vi "Refresh Main Page Listboxes.vi"(6 "Main Page refnums":T3, 8 "error in (no error)":errorcluster, 9 "bitfile listbox":T1, 10 "APU listbox":T1, 11 "Item Ref in":T2 format="%.0x") -> (0 "error out":errorcluster, 1 "bitfile listbox out":T1, 2 "APU listbox out":T1, 3 "Item Ref out":T2=18446744073709551615 format="%.0x")   [LabVIEW 2020, in "Engine Simulation Toolkit System Explorer.lvlib"]
uses:
  Engine Simulation Toolkit System Explorer.lvlib
  Listbox State.ctl
  Main Page refnums.ctl
  <vilib>/NI VeriStand/Custom Device API/Custom Device Item Ref.ctl
  <vilib>/NI VeriStand/Custom Device API/Custom Device API.lvlib
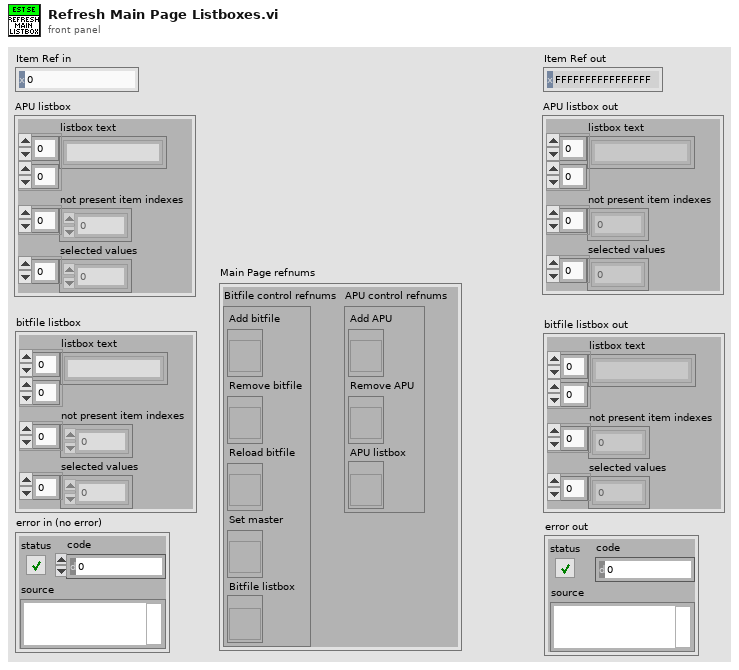
[diagram p1: front panel]
types:
  T1 = typedef "Engine Simulation Toolkit System Explorer.lvlib/Listbox State.ctl" = cluster{"listbox text":string[][], "not present item indexes":i32[], "selected values":i32[]}
  T2 = typedef "Custom Device API.lvlib/Custom Device Item Ref.ctl" = u64
  T3 = typedef "Engine Simulation Toolkit System Explorer.lvlib/Main Page refnums.ctl" = cluster{"Bitfile control refnums":cluster{"Add bitfile":refnum<vi>, "Remove bitfile":refnum<vi>, "Reload bitfile":refnum<vi>, "Set master":refnum<vi>, "Bitfile listbox":refnum<vi>}, "APU control refnums":cluster{"Add APU":refnum<vi>, "Remove APU":refnum<vi>, "APU listbox":refnum<vi>}}
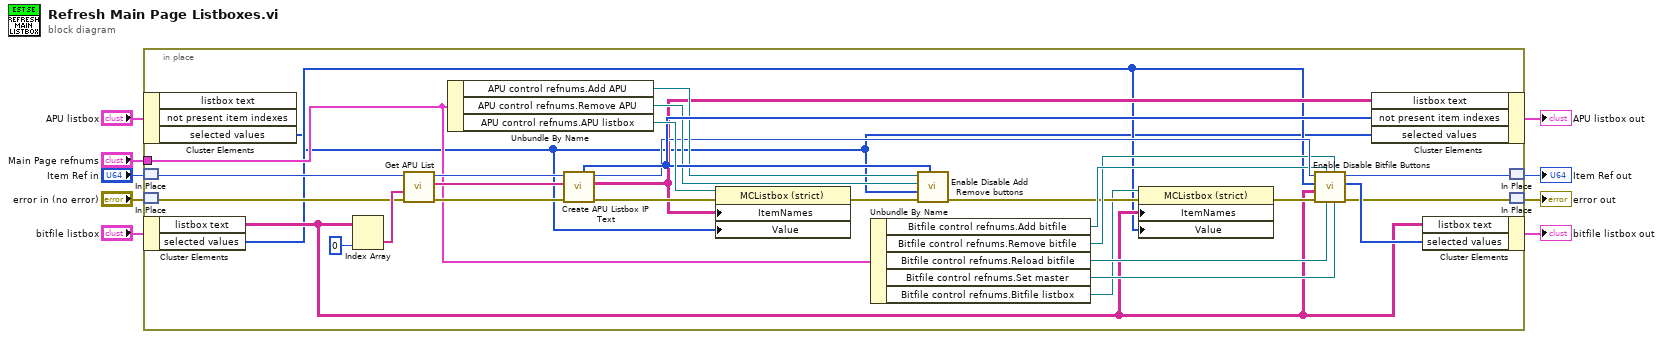
[diagram p0: block diagram]
diagram:
  n1 = in-place {
    in-place-border: "Main Page refnums" -> [w25]
    n2 = in-place-cluster #1("APU listbox") -> ("selected values"=w10:i32[])  [unwired: 2 out]
    n3 = in-place-match #2("Item Ref in") -> (w33:T2)
    n4 = in-place-match #3("error in (no error)") -> (w17:errorcluster)
    n5 = in-place-cluster #4("bitfile listbox") -> ("listbox text"=w12:string[][], "selected values"=w11:i32[])
    n6 = Index Array(array=w12, index (col)=0 ("disabled index (col)")) -> (element=w34:string[])  [unwired: 1 in]
    n7 = call "Get APU List.vi"("error in (no error)"=w17, "rio names"=w34, "Item Ref in"=w33) -> ("error out"=w38:errorcluster, "ips available"=w36:string[], "Item Ref out"=w37:T2)  [unwired: 6 in]
    n8 = Unbundle By Name(w25) -> ("APU control refnums.Add APU"=w28:refnum<vi>, "APU control refnums.Remove APU"=w27:refnum<vi>, "APU control refnums.APU listbox"=w32:refnum<vi>)
    n9 = call "Create APU Listbox IP Text.vi"("error in (no error)"=w38, "ips available"=w36, "Section Ref in"=w37) -> ("error out"=w31:errorcluster, "listbox text"=w16:string[][], "Section Ref out"=w26:T2, "not present item indexes"=w29:i32[])  [unwired: 5 in]
    n10 = property on="Property Node" class="MCListbox (strict)"(reference=w32, error in=w31, "ItemNames"=w16, "Value"=w10) -> (error out=w30:errorcluster)  [unwired: 1 out]
    n11 = Unbundle By Name(w25) -> ("Bitfile control refnums.Add bitfile"=w24:refnum<vi>, "Bitfile control refnums.Remove bitfile"=w23:refnum<vi>, "Bitfile control refnums.Reload bitfile"=w22:refnum<vi>, "Bitfile control refnums.Set master"=w21:refnum<vi>, "Bitfile control refnums.Bitfile listbox"=w13:refnum<vi>)
    n12 = call "Enable Disable Add Remove buttons.vi"("not present item indexes"=w29, "error in (no error)"=w30, "selected items"=w10, "remove button"=w27, "add button"=w28) -> ("error out"=w15:errorcluster)  [unwired: 6 in]
    n13 = property on="Property Node" class="MCListbox (strict)"(reference=w13, error in=w15, "ItemNames"=w12, "Value"=w11) -> (error out=w14:errorcluster)  [unwired: 1 out]
    n14 = call "Enable Disable Bitfile Buttons.vi"("Set Master in"=w21, "Remove in"=w23, "Reload in"=w22, "Add in"=w24, "error in (no error)"=w14, "listbox text"=w12, "Selected Values"=w11, "Item Ref in"=w26) -> ("error out"=w18:errorcluster, "Selected Values"=w20:i32[], "Item Ref out"=w19:T2)  [unwired: 1 in]
    n15 = in-place-cluster #1("listbox text"=w16, "not present item indexes"=w29, "selected values"=w10) -> (→"APU listbox out":T1)
    n16 = in-place-cluster #4("listbox text"=w12, "selected values"=w20) -> (→"bitfile listbox out":T1)
    n17 = in-place-match #2(w19) -> (→"Item Ref out":T2)
    n18 = in-place-match #3(w18) -> (→"error out":errorcluster)
  }
